vi "OA Get Pre Set Mode Names.vi"(11 "pcListOfModes":string) -> (2 "function return":u32, 3 "pcListOfModes out":string)   [LabVIEW 2018, in "AndorSDK.lvlib"]
doc: "EXPNETTYPE unsigned int WINAPI OA_GetPreSetModeNames(char * pcListOfModes);"
uses:
  AndorSDK.lvlib
  ATMCD32D.dll
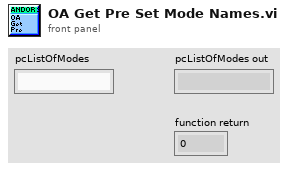
[diagram p1: front panel]
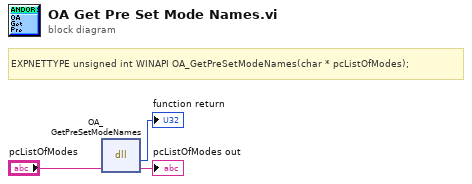
[diagram p0: block diagram]
diagram:
  # "EXPNETTYPE unsigned int WINAPI OA_GetPreSetModeNames(char * pcListOfModes);"
  n1 = dll-call lib="PTH2babs E\nPersönliches02 - Arbeit03-HiwijobsLabviewCodelibANDOR\tAndor SDK\nATMCD32D.*" fn="OA_GetPreSetModeNames"("pcListOfModes"="pcListOfModes") -> (→"function return":u32, "pcListOfModes"=→"pcListOfModes out":string)  [unwired: 3 in, 2 out]
